vi "calculate deltaXbead of tether-use interpolation .vi"() -> ()   [LabVIEW 2014]
uses:
  <vilib>/Analysis/3filter.llb/Savitzky-Golay Filter (DBL).vi
  <vilib>/Utility/file.llb/Read From Spreadsheet File (DBL).vi
  <vilib>/Analysis/NI_AALBase.lvlib
panel:
  in  "side points":i32=6
  in  "Shift":dbl
  out "QPD height for stuckbead (V)":dbl
  out "QPD height for tether (V)":dbl
  in  "T=SG filter\nF=median filter":bool
  in  "T=Fit Left\nF=Fit Right":bool
  out "Stage Step (nm)":dbl
  in  "file path for stuckbead scan data":path
  in  "file path for tether data":path
  out "bead displacement (nm)":dbl[](array[numeric])
  in  "Tab Control":enum32{"Page 1", "Page 2", "Page 4", "Page 3"}(tab)
  out "Stuckbead Scan":T1(graph)
  out "Waveform Graph":dbl[][](graph)
  out "XY Graph 2":T2(graph)
  out "XY Graph":cluster{"Sorted Array":dbl[], dbl[]}[](graph)
  in  "X=T; Y=F":bool
  # "250~450"
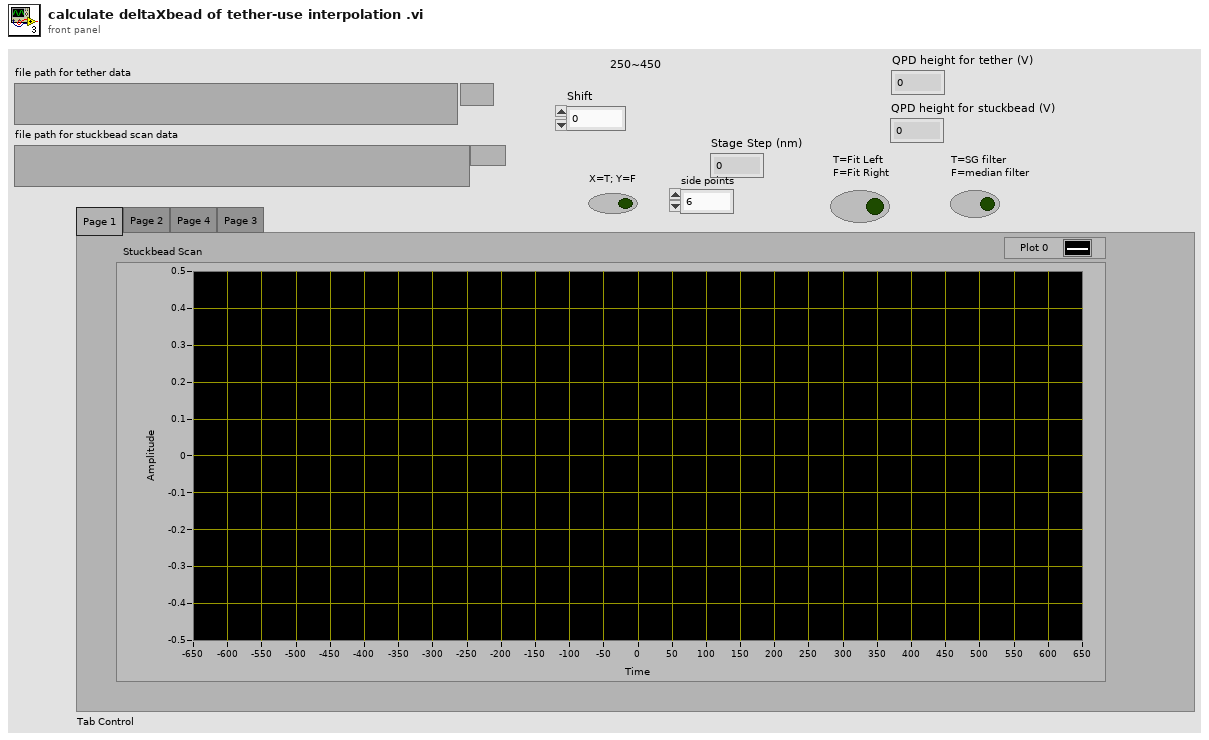
[diagram p1: front panel]
types:
  T1 = cluster{"bead position (nm)":dbl[], "delta Xbead":dbl[]}
  T2 = cluster{"bead displacement (nm)":dbl[], "Filtered X":dbl[]}
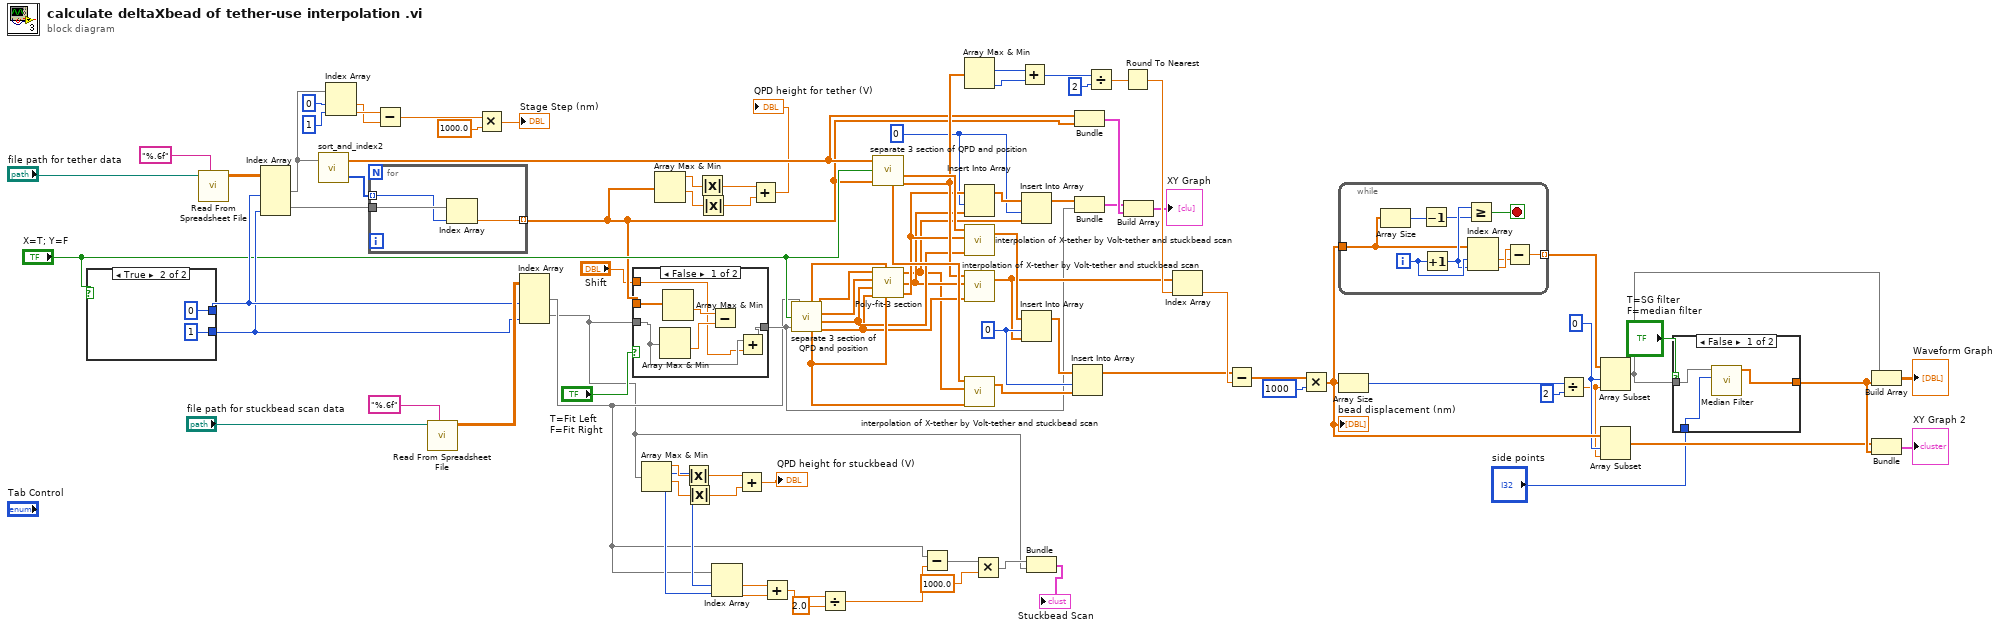
[diagram p0: block diagram]
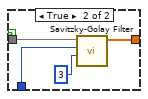
[diagram p2: hidden frame]
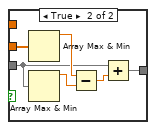
[diagram p3: hidden frame]
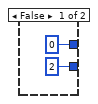
[diagram p4: hidden frame]
diagram:
  w41 = 0 ("index")
  w52 = 0 ("index")
  w71 = 0 ("index")
  n1 = case shown="True" "X=T; Y=F" {
    tunnel: [2 1] -> w88
    tunnel: [0 ("index (row)") 0 ("index (row)")] -> w89
    frame False {
    }
    frame True {
    }
  }
  n2 = call-poly <vilib>:"Read From Spreadsheet File.vi"("format (%.3f)"="%.6f", "file path (dialog if empty)"="file path for tether data") -> ("all rows"=w92:dbl[][])  [unwired: 5 in, 4 out]
  n3 = Index Array(array=w92, index (col) #1=w89, index (col) #2=w88) -> (element #1=w36:dbl[], element #2=w86:dbl[])  [unwired: 2 in]
  n4 = call "sort_and_index2.vi"("Presorted Array"=w36) -> ("Index"=w85:i32[], "Sorted Array"=w65:dbl[])  [unwired: 1 in]
  n5 = Index Array(array=w36, index #1=0 ("index"), index #2=1 ("index")) -> (element #1=w32:dbl, element #2=w33:dbl)
  n6 = for {
    tunnel: w86 -> [w100]
    tunnel: w85 -> [w99] mode=indexing
    tunnel: [w98] -> w26 mode=indexing
    n7 = Index Array(array=w100, index=w99) -> (element=w98:dbl)
  }
  n8 = Subtract(x=w33, y=w32) -> (x-y=w31:dbl)
  n9 = call-poly <vilib>:"Read From Spreadsheet File.vi"("format (%.3f)"="%.6f", "file path (dialog if empty)"="file path for stuckbead scan data") -> ("all rows"=w90:dbl[][])  [unwired: 5 in, 4 out]
  n10 = Multiply(x=w31, y=1000.0) -> (x*y=→"Stage Step (nm)":dbl)
  n11 = Index Array(array=w90, index (col) #1=w89, index (col) #2=w88) -> (element #1=w9:dbl[], element #2=w4:dbl[])  [unwired: 2 in]
  n12 = case shown="False" "T=Fit Left\nF=Fit Right" {
    tunnel: w4 -> [w103 w110]
    tunnel: [w102 w109] -> w66
    tunnel: w26 -> [w106 w108]
    tunnel: "Shift" -> [w101 _]
    frame False {
      n13 = Array Max & Min(array=w103) -> (min value=w104:dbl)  [unwired: 3 out]
      n14 = Array Max & Min(array=w106) -> (min value=w105:dbl)  [unwired: 3 out]
      n15 = Subtract(x=w105, y=w104) -> ()  [unwired: 1 out]
      n16 = Add(x=w103, y=w101) -> (x+y=w102:dbl[])
    }
    frame True {
      n17 = Array Max & Min(array=w108) -> (max value=w112:dbl)  [unwired: 3 out]
      n18 = Array Max & Min(array=w110) -> (max value=w111:dbl)  [unwired: 3 out]
      n19 = Subtract(x=w112, y=w111) -> (x-y=w107:dbl)
      n20 = Add(x=w110, y=w107) -> (x+y=w109:dbl[])
    }
  }
  n21 = Array Max & Min(array=w4) -> (max value=w20:dbl, max index (indices)=w15:i32, min value=w19:dbl, min index (indices)=w14:i32)
  n22 = Array Max & Min(array=w26) -> (max value=w25:dbl, min value=w24:dbl)  [unwired: 2 out]
  n23 = Absolute Value(x=w20) -> (abs(x)=w18:dbl)
  n24 = Absolute Value(x=w19) -> (abs(x)=w17:dbl)
  n25 = Absolute Value(x=w25) -> (abs(x)=w23:dbl)
  n26 = Absolute Value(x=w24) -> (abs(x)=w22:dbl)
  n27 = Index Array(array=w9, index #1=w15, index #2=w14) -> (element #1=w13:dbl, element #2=w12:dbl)
  n28 = Add(x=w18, y=w17) -> (x+y=→"QPD height for stuckbead (V)":dbl)
  n29 = Add(x=w23, y=w22) -> (x+y=→"QPD height for tether (V)":dbl)
  n30 = Add(x=w13, y=w12) -> (x+y=w11:dbl)
  n31 = call "separate 3 section of QPD and position.vi"("QPD signal (V)"=w66, "X=T; Y=F"="X=T; Y=F", "stage position (um)"=w9) -> ("2nd section of QPD (V)"=w56:dbl[], "1st section of QPD (V)"=w60:dbl[], "3rd section of QPD (V)"=w57:dbl[], "3rd section of position (um)"=w58:dbl[], "1st section of position (um)"=w61:dbl[], "2nd section of position (um)"=w59:dbl[])
  n32 = Divide(x=w11, y=2.0) -> (x/y=w8:dbl)
  n33 = call "separate 3 section of QPD and position.vi"("QPD signal (V)"=w26, "X=T; Y=F"="X=T; Y=F", "stage position (um)"=w65) -> ("2nd section of QPD (V)"=w82:dbl[], "1st section of QPD (V)"=w84:dbl[], "3rd section of QPD (V)"=w83:dbl[])  [unwired: 3 out]
  n34 = call "Poly-fit-3 section.vi"("2nd stage position (um)"=w59, "1st stage position (um)"=w61, "3rd stage position (um)"=w58, "3rd QPD signal (V)"=w57, "1st QPD signal (V)"=w60, "2nd QPD signal (V)"=w56) -> ("1st Best stage position"=w51:dbl[], "2nd Best stage position"=w54:dbl[], "3rd Best stage position"=w55:dbl[])
  n35 = Subtract(x=w9, y=w8) -> (x-y=w7:dbl[])
  n36 = Array Max & Min(array=w82) -> (max index (indices)=w81:i32, min index (indices)=w79:i32)  [unwired: 2 out]
  n37 = Insert Into Array(array=w55, index=w52, new element=w54) -> (w53:dbl[])
  n38 = call "interpolation of X-tether by Volt-tether and stuckbead scan.vi"("stuckbead-QPD (V)"=w57, "stuckbead-stage position (um)"=w55, "tether-QPD (V)"=w83) -> ("Xt-interpolated (um)"=w72:dbl[])  [unwired: 2 in]
  n39 = call "interpolation of X-tether by Volt-tether and stuckbead scan.vi"("stuckbead-QPD (V)"=w56, "stuckbead-stage position (um)"=w54, "tether-QPD (V)"=w82) -> ("Xt-interpolated (um)"=w68:dbl[])  [unwired: 2 in]
  n40 = call "interpolation of X-tether by Volt-tether and stuckbead scan.vi"("stuckbead-QPD (V)"=w60, "stuckbead-stage position (um)"=w51, "tether-QPD (V)"=w84) -> ("Xt-interpolated (um)"=w70:dbl[])  [unwired: 2 in]
  n41 = Multiply(x=w7, y=1000.0) -> (x*y=w5:dbl[])
  n42 = Add(x=w81, y=w79) -> (x+y=w80:i32)
  n43 = Insert Into Array(array=w53, index=w52, new element=w51) -> (w49:dbl[])
  n44 = Insert Into Array(array=w72, index=w71, new element=w68) -> (w69:dbl[])
  n45 = Bundle(w5, "all rows"=w4) -> (→"Stuckbead Scan":cluster{dbl[], "all rows":dbl[]})  [unwired: 1 in]
  n46 = Insert Into Array(array=w69, index=w71, new element=w70) -> (w67:dbl[])
  n47 = Bundle("Sorted Array"=w65, w26) -> (w64:cluster{"Sorted Array":dbl[], dbl[]})  [unwired: 1 in]
  n48 = Bundle("3rd Best stage position"=w49, w66) -> (w50:cluster{"3rd Best stage position":dbl[], dbl[]})  [unwired: 1 in]
  n49 = Divide(x=w80, y=2) -> (x/y=w77:dbl)
  n50 = Round To Nearest(number=w77) -> (nearest integer value=w76:dbl)
  n51 = Build Array(w50, w64) -> (→"XY Graph":cluster{"Sorted Array":dbl[], dbl[]}[])
  n52 = Index Array(array=w68, index=w76) -> (element=w75:dbl)
  n53 = Subtract(x=w67, y=w75) -> (x-y=w74:dbl[])
  n54 = Multiply(x=w74, y=1000) -> (x*y=w46:dbl[])
  "bead displacement (nm)" <- w46
  n55 = while {
    tunnel: w46 -> [w113]
    tunnel: [w118] -> w42 mode=indexing
    i -> [w121]
    stop <- w114 stop-if-true
    n56 = Array Size(array=w113) -> (size(s)=w116:i32)
    n57 = Decrement(x=w116) -> (x-1=w115:i32)
    n58 = Increment(x=w121) -> (x+1=w117:i32)
    n59 = Greater Or Equal?(x=w117, y=w115) -> (x >= y?=w114:bool)
    n60 = Index Array(array=w113, index #1=w121, index #2=w117) -> (element #1=w119:dbl, element #2=w120:dbl)
    n61 = Subtract(x=w120, y=w119) -> (x-y=w118:dbl)
  }
  n62 = Array Size(array=w46) -> (size(s)=w45:i32)
  n63 = Divide(x=w45, y=2) -> (x/y=w40:dbl)
  n64 = Array Subset(array=w42, index=w41, length=w40) -> (w39:dbl[])
  n65 = Array Subset(array=w46, index=w41, length=w40) -> (w43:dbl[])
  n66 = case shown="False" "T=SG filter\nF=median filter" {
    tunnel: [w123 w127] -> w48
    tunnel: w39 -> [w124 w126]
    tunnel: "side points" -> [w122 w125]
    frame False {
      n67 = call <vilib>:"Median Filter.vi"("left rank"=w122, "X"=w124) -> ("Filtered X"=w123:dbl[])  [unwired: 8 in, 1 out]
    }
    frame True {
      n68 = call-poly <vilib>:"Savitzky-Golay Filter.vi"("polynomial order"=3, "side points"=w125, "X"=w126) -> ("Filtered X"=w127:dbl[])  [unwired: 7 in, 1 out]
    }
  }
  n69 = Build Array(w39, w48) -> (→"Waveform Graph":dbl[][])
  n70 = Bundle(w43, "Filtered X"=w48) -> (→"XY Graph 2":cluster{dbl[], "Filtered X":dbl[]})  [unwired: 1 in]
